vi "Servos.vi"() -> ()   [LabVIEW 2018]
panel:
  in  "Servo B":dbl(slide) scale=-200.0..200.0
  in  "Servo A":dbl(slide) scale=-200.0..200.0
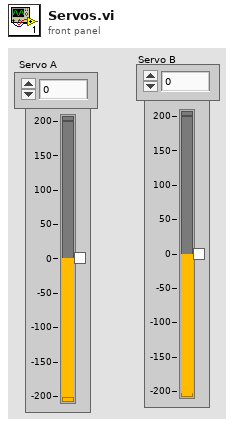
[diagram p1: front panel]
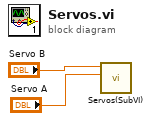
[diagram p0: block diagram]
diagram:
  n1 = call "Servos(SubVI).vi"(10:"Servo A", 11:"Servo B") -> ()  [unwired: 10 in]
